vi "Comms Snippet.vi"   [LabVIEW 2020]
uses:
  NHMFL_Core/Libraries/Red Pitaya/RP Core/Red Pitaya Transceiver Driver/Spectrum Configuration.ctl
  <vilib>/ActorFramework/Actor/Actor.lvclass
  Template Module Messages/Message Nested Object Msg/Message Nested Object Msg.lvclass
  Template Module Messages/Write FP Control Msg/Write FP Control Msg.lvclass
  C:/Program Files/National Instruments/LabVIEW 2020/vi.lib/ActorFramework/Message/Message.lvclass
  C:/GitHub/LabActor/Template Module Messages/Write FP Control Msg/Write FP Control Msg.lvclass
types:
  T1 = typedef "Spectrum Configuration.ctl" = cluster{"Start frequency":dbl, "End frequency":dbl, "Coarse step":dbl, "Step duration":dbl, "Red Pitaya address":string, "Open plot \non start":bool, "Regions width":dbl, "Fine step":dbl, "Pause between scans":dbl, "Clear rgs on start":bool, "Output amplitude":dbl, "Append measurements":string[]}
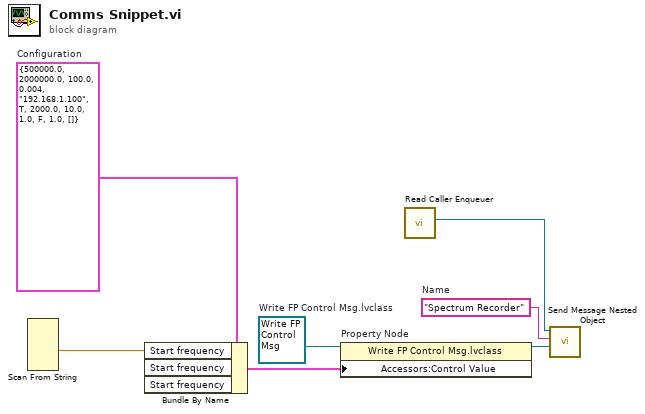
[diagram p0: block diagram]
diagram:
  w1 = "Spectrum Recorder"  # Name
  w5 = refnum<class "Write FP Control Msg.lvclass"> refnum  # Write FP Control Msg.lvclass
  w7 = T1 {"Start frequency"=500000.0, "End frequency"=2000000.0, "Coarse step"=100.0, "Step duration"=0.004, "Red Pitaya address"="192.168.1.100", "Open plot \non start"=TRUE, "Regions width"=2000.0, "Fine step"=10.0, "Pause between scans"=1.0, "Clear rgs on start"=FALSE, "Output amplitude"=1.0, "Append measurements"=[]}  # Configuration
  n1 = Scan From String "Scan From String"() -> (output 1=w6:dbl)  [unwired: 9 in, 3 out]
  n2 = Bundle By Name "Bundle By Name"(cluster=w7, "Start frequency"=w6) -> (w4:T1)  [unwired: 2 in]
  n3 = property on="Property Node" class="Write FP Control Msg.lvclass"(reference=w5, "Accessors:Control Value"=w4) -> (reference out=w2:refnum<class "Write FP Control Msg.lvclass">)  [unwired: 1 in, 1 out]
  n4 = call <vilib>:"Read Caller Enqueuer.vi"() -> ("Caller Enqueuer"=w3:refnum<class "Message Enqueuer.lvclass">)  [unwired: 11 in]
  n5 = call "Send Message Nested Object.vi"("Message"=w2, "Name"=w1, "Message Enqueuer"=w3) -> ()  [unwired: 7 in, 2 out]
